vi "Get Request Type.vi"(8 "error in (no error)":errorcluster, 11 "GetVersion in":refnum<class "GetVersion.lvclass">) -> (0 "error out":errorcluster, 2 "Request Type":string, 3 "GetVersion out":refnum<class "GetVersion.lvclass">)   [LabVIEW 2022 SP3, in "obs-websocket-lv.lvlib" / "GetVersion.lvclass"]
uses:
  GetVersion.lvclass
  GetVersion.lvclass/GetVersion.ctl
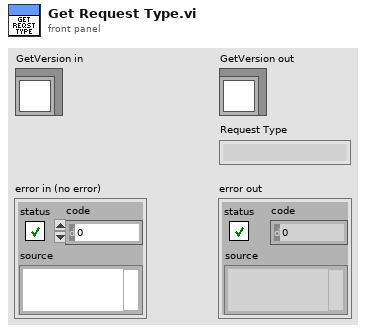
[diagram p1: front panel]
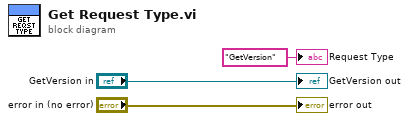
[diagram p0: block diagram]
diagram:
  "error out" <- "error in (no error)"
  "GetVersion out" <- "GetVersion in"
  "Request Type" <- "GetVersion" ("Request Type")
